vi "External Message Handler.vi"(8 "error in (no error)":errorcluster, 11 "AssertEngine in":refnum<class "AssertEngine.lvclass">) -> (0 "error out":errorcluster)   [LabVIEW 2016, in "AssertEngine.lvlib" / "AssertEngine.lvclass"]
doc: "Helper loop vi to accept messages coming in from the external message queue and pass them correctly into the main Assert Engine"
uses:
  AssertEngine.lvclass
  C:/Program Files/National Instruments/LabVIEW 2016/vi.lib/ActorFramework/Actor/Actor.lvclass
  <vilib>/ActorFramework/Actor/Actor.lvclass/Actor.ctl
  <vilib>/ActorFramework/Message Enqueuer/Message Enqueuer.lvclass/Message Enqueuer.ctl
  AssertEngine.lvclass/AssertEngine.ctl
  <vilib>/ActorFramework/Report Error Msg/Report Error Msg.lvclass/Report Error Msg.ctl
  <vilib>/ActorFramework/Message Enqueuer/Init from Existing Queue.vi
  <vilib>/ActorFramework/Message Enqueuer/Enqueue.vi
  <vilib>/ActorFramework/Report Error Msg/Report Error Msg.lvclass
  C:/Program Files/National Instruments/LabVIEW 2016/vi.lib/ActorFramework/Message/Message.lvclass
  <vilib>/ActorFramework/Message Priority Queue/Priority Enqueue.vi
  <vilib>/ActorFramework/Message Enqueuer/Message Enqueuer.lvclass
  External Message Queue/Classes/External Msg.lvclass
  <vilib>/ActorFramework/Actor/Actor.lvclass
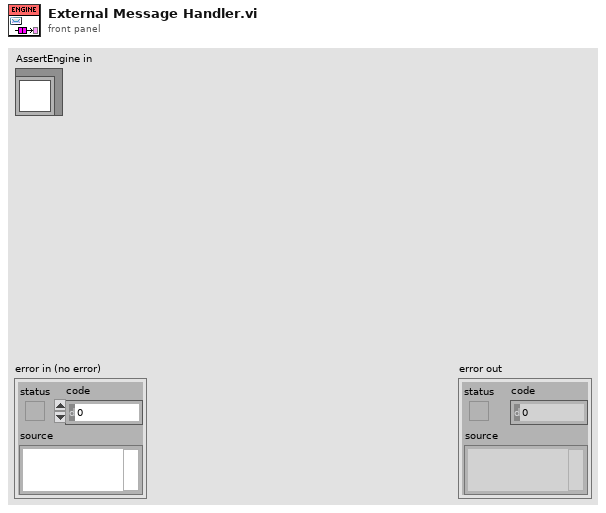
[diagram p1: front panel]
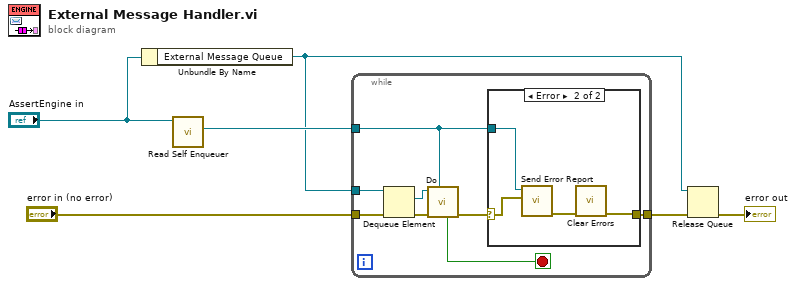
[diagram p0: block diagram]
diagram:
  n1 = Unbundle By Name("AssertEngine in") -> ("External Message Queue"=w1:refnum<queue>)
  n2 = call <vilib>:"Read Self Enqueuer.vi"("Actor"="AssertEngine in") -> ("Self Enqueuer"=w3:refnum<class "Message Enqueuer.lvclass">)  [unwired: 10 in]
  n3 = while {
    tunnel: w1 -> [w14]
    tunnel: "error in (no error)" -> [w13]
    tunnel: [w8] -> w5
    tunnel: w3 -> [w7]
    stop <- w9 stop-if-true
    n4 = Dequeue Element(queue=w14, error in (no error)=w13) -> (element=w12:refnum<class "External Msg.lvclass">, error out=w11:errorcluster)  [unwired: 1 in, 2 out]
    n5 = call-dynamic "Do.vi"("Engine Enqueuer"=w7, "error in (no error)"=w11, "External Msg in"=w12) -> ("error out"=w10:errorcluster, "Stop"=w9:bool)  [unwired: 7 in]
    n6 = case shown="Error" w10 {
      selector: w10 -> [w15 w19]
      tunnel: [w15 w17] -> w8
      tunnel: w7 -> [_ w16]
      frame No Error {
      }
      frame Error {
        n7 = call <vilib>:"Send Error Report.vi"("Error From Sender"=w19, "Message Enqueuer"=w16) -> ("error out"=w18:errorcluster)  [unwired: 9 in]
        n8 = call <vilib>:"Clear Errors.vi"("error in (no error)"=w18) -> ("error out"=w17:errorcluster)  [unwired: 5 in, 1 out]
      }
    }
  }
  n9 = Release Queue(queue=w1, error in (no error)=w5) -> (error out=→"error out":errorcluster)  [unwired: 1 in, 2 out]
